vi "Lookup Implementation.vi"(8 "error in (no error)":errorcluster, 10 "Implementation Tag":string, 11 "Malleable VI Type in":refnum<class "Malleable VI Type.lvclass">) -> (0 "error out":errorcluster, 2 "Found?":bool, 3 "Malleable VI Type out":refnum<class "Malleable VI Type.lvclass">)   [LabVIEW 2020, in "Peek Window.lvlib" / "Malleable VI Type.lvclass"]
uses:
  Malleable VI Type.lvclass
  D:/Code/VI-Peek/source/Peek Window/VI Types/Standard VI Type/Standard VI Type.lvclass
  Selected Implementation Enum.ctl
  Implementation VI Type/Implementation VI Type.lvclass
  Malleable VI Type.lvclass/Malleable VI Type.ctl
  Standard VI Type/Standard VI Type.lvclass/Standard VI Type.ctl
  Standard VI Type/Read VI Refnum.vi
  Standard VI Type/Read Full Qualified Name.vi
  Standard VI Type/Write VI Refnum.vi
  Standard VI Type/Write Full Qualified Name.vi
  <vilib>/Utility/error.llb/Error Cluster From Error Code.vi
  <vilib>/ErrorRing/Error Ring.xnode
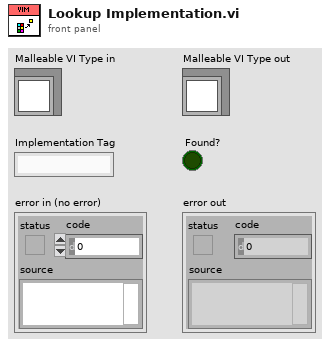
[diagram p1: front panel]
types:
  T1 = typedef "Peek Window.lvlib/Malleable VI Type.lvclass/Selected Implementation Enum.ctl" = enum16{"Actual", "Instance"}
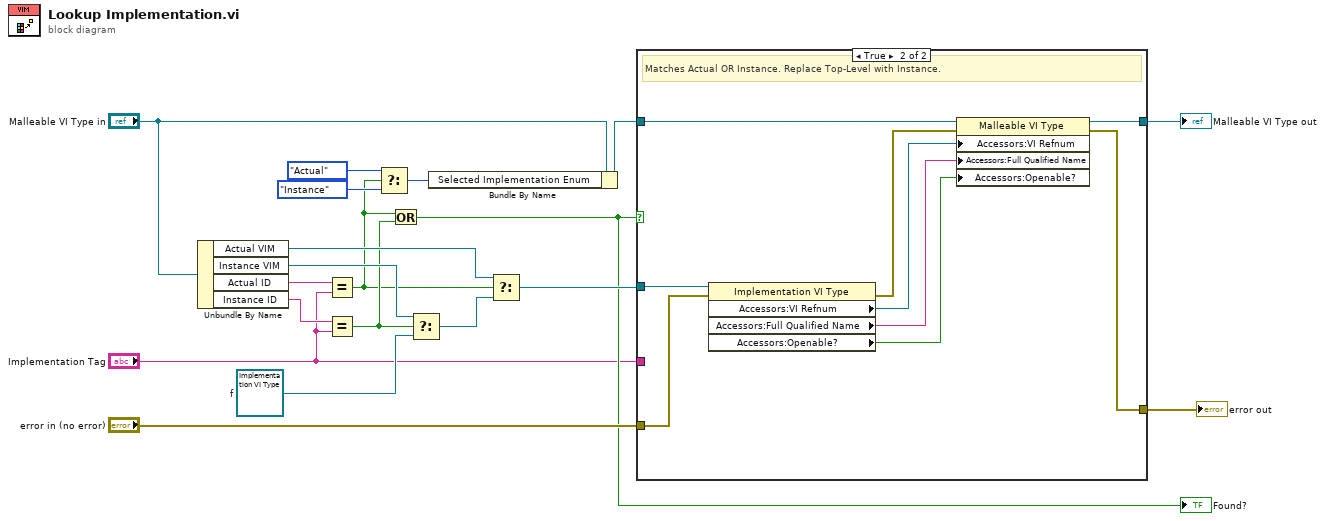
[diagram p0: block diagram]
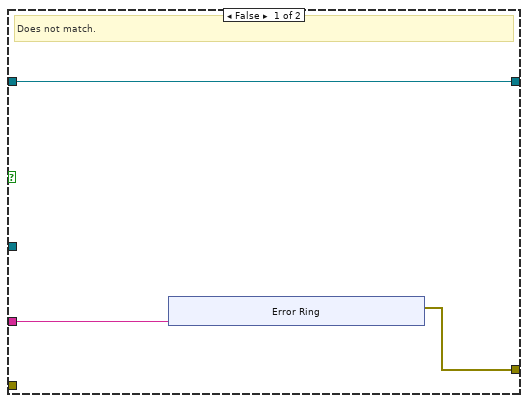
[diagram p2: hidden frame]
diagram:
  w10 = refnum<class "Implementation VI Type.lvclass"> refnum  # f
  n1 = Unbundle By Name("Malleable VI Type in") -> ("Actual VIM"=w14:refnum<class "Implementation VI Type.lvclass">, "Instance VIM"=w12:refnum<class "Implementation VI Type.lvclass">, "Actual ID"=w15:string, "Instance ID"=w13:string)
  n2 = Equal?(x=w15, y="Implementation Tag") -> (x = y?=w8:bool)
  n3 = Equal?(x=w13, y="Implementation Tag") -> (x = y?=w9:bool)
  n4 = Select(t=Selected_Implementation_Enum."Actual", s=w8, f=Selected_Implementation_Enum."Instance") -> (s? t:f=w16:T1)
  n5 = Or(x=w8, y=w9) -> (x .or. y?=w2:bool)
  "Found?" <- w2
  n6 = Select(t=w12, s=w9, f=w10) -> (s? t:f=w11:refnum<class "Implementation VI Type.lvclass">)
  n7 = Bundle By Name(cluster="Malleable VI Type in", "Selected Implementation Enum"=w16) -> (w6:refnum<class "Malleable VI Type.lvclass">)
  n8 = Select(t=w14, s=w8, f=w11) -> (s? t:f=w3:refnum<class "Implementation VI Type.lvclass">)
  n9 = case shown="True" w2 {
    tunnel: [w22 w35] -> w7
    tunnel: w6 -> [w22 w34]
    tunnel: [w20 w33] -> w5
    tunnel: "error in (no error)" -> [_ w32]
    tunnel: w3 -> [_ w31]
    tunnel: "Implementation Tag" -> [w21 _]
    frame False {
      # "Does not match."
      n10 = xnode "Error Ring"("parameter 0"=w21) -> ("error out"=w20:errorcluster)
    }
    frame True {
      # "Matches Actual OR Instance. Replace Top-Level with Instance."
      n11 = property class="Implementation VI Type"(reference=w31, error in=w32) -> (error out=w38:errorcluster, "Accessors:VI Refnum"=w37:refnum<vi>, "Accessors:Full Qualified Name"=w36:string, "Accessors:Openable?"=w30:bool)  [unwired: 1 out]
      n12 = property class="Malleable VI Type"(reference=w34, error in=w38, "Accessors:VI Refnum"=w37, "Accessors:Full Qualified Name"=w36, "Accessors:Openable?"=w30) -> (reference out=w35:refnum<class "Malleable VI Type.lvclass">, error out=w33:errorcluster)
    }
  }
  "error out" <- w5
  "Malleable VI Type out" <- w7
